vi "Do.vi"(8 "error in":errorcluster, 10 "Actor in":refnum<class "Actor.lvclass">, 11 "Change Laser Enable State":refnum<class "Change Laser Enable State.lvclass">) -> (0 "error out":errorcluster, 2 "Actor out":refnum<class "Actor.lvclass">)   [LabVIEW 2018, in "eCRDS Library.lvlib" / "Change Laser Enable State.lvclass"]
doc: "(<B>Filename</B>: Actor Framework.lvlib:Message.lvclass:Do.vi)\n\nDefines what a message does when it is received by an actor. Generally, a message instructs an actor to invoke one of its methods. By default, this method does nothing. A child class must override it to define behavior. Create a child class by using the Actor Framework Message Maker dialog box."
uses:
  Change Laser Enable State.lvclass
  Instr Actor/Instr Actor.lvclass
  reusable/Session APIs/CVT/CVT.lvclass
  Commands/Change Laser Enable State/Laser Enable CMD.lvclass
  reusable/Command/Command.lvclass
  C:/Users/Labview/Documents/exscalabar_server/SuperActor/SuperActor.lvclass
  C:/Program Files (x86)/National Instruments/LabVIEW 2018/vi.lib/ActorFramework/Actor/Actor.lvclass
  C:/Users/Labview/Documents/exscalabar_server/reusable/Command/Command.lvclass
  <vilib>/ActorFramework/Actor/Actor.lvclass
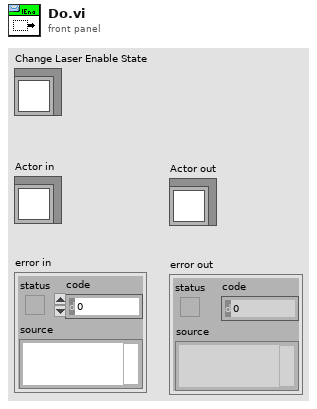
[diagram p1: front panel]
types:
  T1 = typedef "Session - Root.lvclass/Session Handle.ctl" = refnum<data-value>
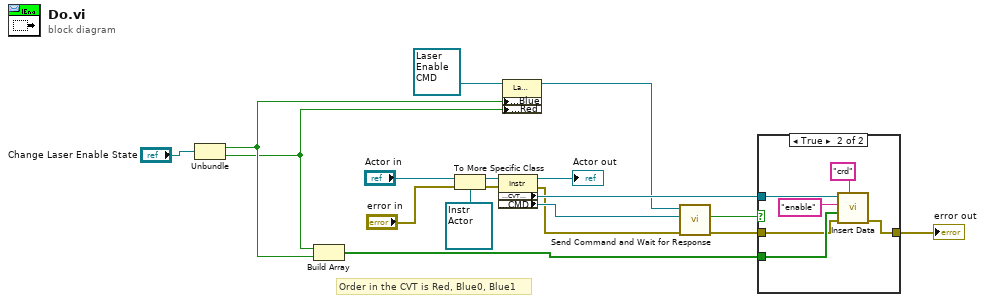
[diagram p0: block diagram]
diagram:
  # "Order in the CVT is Red, Blue0, Blue1"
  n1 = Unbundle("Change Laser Enable State") -> (w7:bool, w6:bool)
  n2 = Build Array(w6, w7) -> (w11:bool[])
  n3 = To More Specific Class(target class=refnum<class "Instr Actor.lvclass"> refnum ("Instrument Lib:Instr"), reference="Actor in", error in="error in") -> (specific class reference=w14:refnum<class "Instr Actor.lvclass">, error out=w9:errorcluster)
  n4 = property class="Instr"(reference=w14, error in=w9) -> (reference out=→"Actor out":refnum<class "Instr Actor.lvclass">, error out=w1:errorcluster, "Accessors:CVT Session"=w12:T1, "Accessors:CMD"=w4:refnum<queue>)
  n5 = property class="Laser Enable CMD.lvclass"(reference=refnum<class "Laser Enable CMD.lvclass"> refnum ("eCRDS Library.lvlib:Laser Enable CMD.lvclass"), "Accessors:Blue"=w7, "Accessors:Red"=w6) -> (reference out=w5:refnum<class "Laser Enable CMD.lvclass">)  [unwired: 1 in, 1 out]
  n6 = call "Send Command and Wait for Response.vi"("error in"=w1, "cmd queue"=w4, "CMD in"=w5) -> ("error out"=w2:errorcluster, "cmd good?"=w3:bool)  [unwired: 6 in, 1 out]
  n7 = case shown="True" w3 {
    tunnel: w12 -> [_ w25]
    tunnel: w11 -> [_ w22]
    tunnel: [w19 w21] -> w10
    tunnel: w2 -> [w19 w20]
    frame False {
    }
    frame True {
      n8 = call "Insert Data.vi"("Group"="crd", "error in"=w20, "Data"=w22, "tag"="enable", "CVT Session In"=w25) -> ("error out"=w21:errorcluster)  [unwired: 5 in, 1 out]
    }
  }
  "error out" <- w10
